vi "pmu_Phasor Measurement.vi"(0 "reporting raw data":T1, 2 "reset? (F)":bool, 5 "buffered zero-crossing frequencies":T2, 9 "system info in":refnum<class "PMU System Info.lvclass">, 11 "error in (no error)":errorcluster) -> (3 "physical phasors":csg[](array[numeric]), 4 "reporting phasors":csg[](array[numeric]), 6 "reporting frequency":sgl, 8 "reporting df/dt":sgl, 10 "system info out":refnum<class "PMU System Info.lvclass">, 15 "error out":errorcluster)   [LabVIEW 2013, in "NI_EP_PMU.lvlib"]
doc: "Calculates <b>phasors</b> and measures the <b>frequency</b> and the rate of change of frequency, <b>df/dt</b>, of input waveforms, according to IEEE Std C37.118."
uses:
  <vilib>/addons/Electrical Power/PMU/NI_EP_PMU.lvlib
  <vilib>/addons/Electrical Power/PMU/Common/Classes/PMU System Info/PMU System Info.lvclass
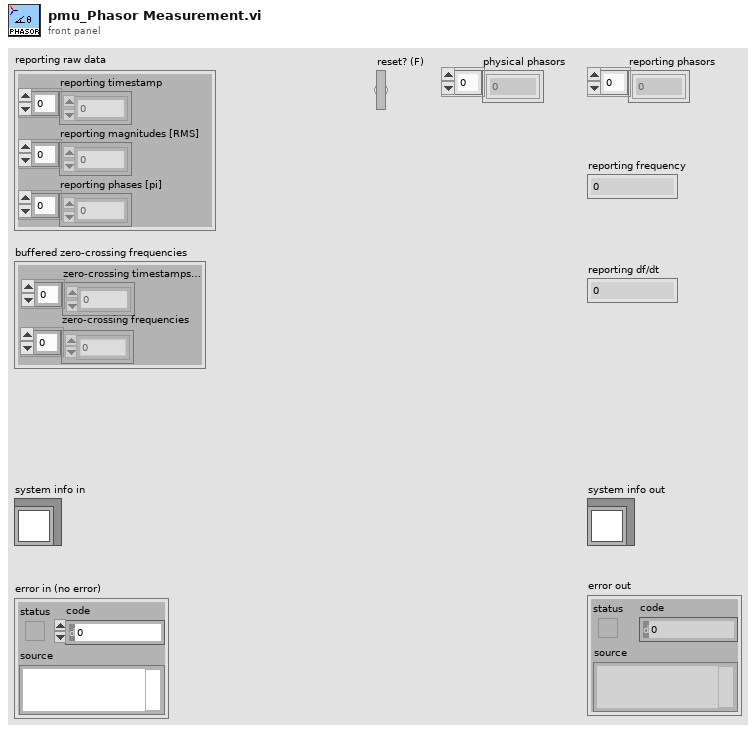
[diagram p1: front panel]
types:
  T1 = cluster{"reporting timestamp":dbl[], "reporting magnitudes [RMS]":dbl[], "reporting phases [pi]":dbl[]}
  T2 = cluster{"zero-crossing timestamps [s]":dbl[], "zero-crossing frequencies":dbl[]}
  T3 = typedef "NI_EP_PMU.lvlib/pmu_CFG Class.ctl" = cluster{"station name":string, "PMU ID":u16, "time base":u32, "nominal frequency":enum16{"50 Hz", "60 Hz"}, "reporting rate":i16, "phasor number":u16, "analog number":u16, "digital number":u16, "channel names":string[], "phasor units":u32[], "analog units":u32[], "digital units":u32[], "data format":u16, "number of PMUs":u16}
  T4 = typedef "LVDateTimeRec.ctl" = cluster{"fractional second":dbl, "second":i32, "minute":i32, "hour":i32, "day of month":i32, "month":i32, "year":i32, "day of week":i32, "day of year":i32, "DST":i32}
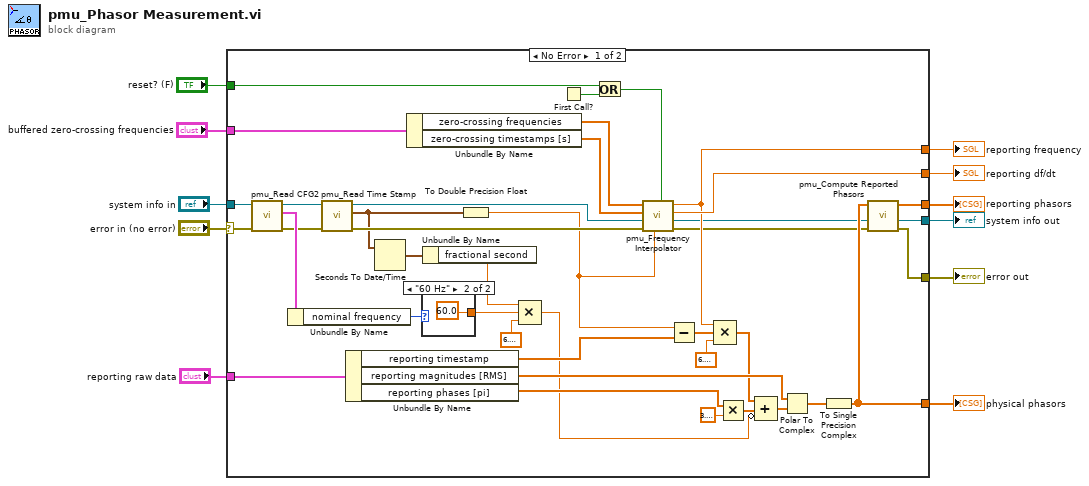
[diagram p0: block diagram]
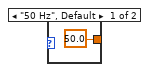
[diagram p2: hidden frame]
diagram:
  n1 = case shown="No Error" "error in (no error)" {
    selector: "error in (no error)" -> [w30 w55]
    tunnel: [w50 w55] -> w10
    tunnel: "system info in" -> [w31 w54]
    tunnel: [w51 w54] -> w8
    tunnel: [w41 _] -> w7
    tunnel: [w35 _] -> w6
    tunnel: [w49 _] -> w5
    tunnel: "reset? (F)" -> [w48 _]
    tunnel: [w45 _] -> w3
    tunnel: "buffered zero-crossing frequencies" -> [w44 _]
    tunnel: "reporting raw data" -> [w37 _]
    frame No Error {
      n2 = call <vilib>:"pmu_Read CFG2.vi"("error in (no error)"=w30, "system info in"=w31) -> ("error out"=w29:errorcluster, "CFG-2"=w32:T3, "system info out"=w28:refnum<class "PMU System Info.lvclass">)  [unwired: 7 in]
      n3 = Unbundle By Name(w32) -> ("nominal frequency"=w26:enum16{"50 Hz", "60 Hz"})
      n4 = call <vilib>:"pmu_Read Time Stamp.vi"("error in (no error)"=w29, "system info in"=w28) -> ("error out"=w34:errorcluster, "time stamp"=w22:timestamp, "system info out"=w19:refnum<class "PMU System Info.lvclass">)  [unwired: 7 in]
      n5 = Unbundle By Name(w37) -> ("reporting timestamp"=w38:dbl[], "reporting magnitudes [RMS]"=w39:dbl[], "reporting phases [pi]"=w40:dbl[])
      n6 = Seconds To Date/Time(time stamp (now)=w22) -> (date time rec=w21:T4)  [unwired: 1 in]
      n7 = Unbundle By Name(w44) -> ("zero-crossing frequencies"=w42:dbl[], "zero-crossing timestamps [s]"=w43:dbl[])
      n8 = case shown="\"60 Hz\"" w26 {
        tunnel: [sgl 50.0 ("value") sgl 60.0 ("value")] -> w23
        frame "50 Hz", Default {
        }
        frame "60 Hz" {
        }
      }
      n9 = Unbundle By Name(w21) -> ("fractional second"=w20:dbl)
      n10 = To Double Precision Float(number=w22) -> (double precision float=w24:dbl)
      n11 = Compound Arithmetic op=MULTIPLY(w20, w23, sgl 6.2831855 ("value")) -> (w27:dbl)
      n12 = First Call?() -> (First Call?: T/F=w47:bool)
      n13 = Or(x=w48, y=w47) -> (x .or. y?=w46:bool)
      n14 = call <vilib>:"pmu_Frequency Interpolator.vi"("reset? (F)"=w46, "reported time"=w24, "error in (no error)"=w34, "PMU system info in"=w19, "timestamps"=w43, "frequencies"=w42) -> ("error out"=w33:errorcluster, "PMU system info out"=w18:refnum<class "PMU System Info.lvclass">, "df/dt"=w45:sgl, "frequency"=w41:sgl)  [unwired: 2 in]
      n15 = Subtract(x=w24, y=w38) -> (x-y=w15:dbl[])
      n16 = Compound Arithmetic op=MULTIPLY(w41, w15, sgl 6.2831855 ("value")) -> (w14:dbl[])
      n17 = Multiply(x=w40, y=3.141592653589793) -> (x*y=w13:dbl[])
      n18 = Compound Arithmetic op=ADD(w14, w13, invert w27) -> (w12:dbl[])
      n19 = Polar To Complex(1:w12, 2:w39) -> (0:w36:cdb[])
      n20 = To Single Precision Complex(1:w36) -> (0:w35:csg[])
      n21 = call <vilib>:"pmu_Compute Reported Phasors.vi"("error in (no error)"=w33, "PMU system info in"=w18, "physical channel phasors"=w35) -> ("error out"=w50:errorcluster, "PMU system info out"=w51:refnum<class "PMU System Info.lvclass">, "reported phasors"=w49:csg[])  [unwired: 6 in]
    }
    frame Error {
    }
  }
  "error out" <- w10
  "reporting frequency" <- w7
  "system info out" <- w8
  "reporting df/dt" <- w3
  "physical phasors" <- w6
  "reporting phasors" <- w5
